vi "LoadDataLog.vi"(3 "entrée d'erreur":errorcluster, 4 "Shoot number to load":i32, 5 "Exp. folder":path) -> (0 "sortie d'erreur":errorcluster, 1 "Header Array":string[](array[string]), 2 "DataLoggingCluster":T1 {"Add. Param. No 2" format="%#_6f"; "Add. Param. No 1" format="%#_6f"; "Wedge Insertion (mm)" format="%#_6f"; "Pulse Duration (fs)" format="%#_6f"; "Parabola Position (um)" format="%#_6f"; "Pulse Energy (mJ)" format="%#_6f"; "Chirp (fs^2)" format="%#_6f"})   [LabVIEW 2014, in "ShhgDataLogging.lvlib"]
uses:
  ShhgDataLogging.lvlib
  DataLoggingCluster.ctl
panel:
  out "TimeString":string
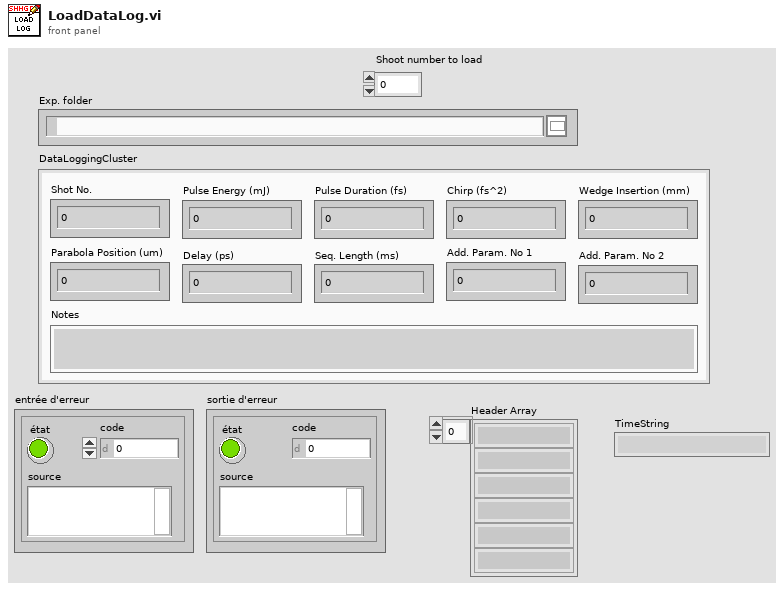
[diagram p1: front panel]
types:
  T1 = typedef "ShhgDataLogging.lvlib/DataLoggingCluster.ctl" = cluster{"Shot No. ":u32, "Pulse Energy (mJ)":dbl, "Pulse Duration (fs)":dbl, "Chirp (fs^2)":dbl, "Wedge Insertion (mm)":dbl, "Parabola Position (um)":dbl, "Delay (ps)":dbl, "Seq. Length (ms)":dbl, "Add. Param. No 1":dbl, "Add. Param. No 2":dbl, "Notes":string}
  T2 = enum16{"open", "replace", "create", "open or create", "replace or create", "replace or create with confirmation"}
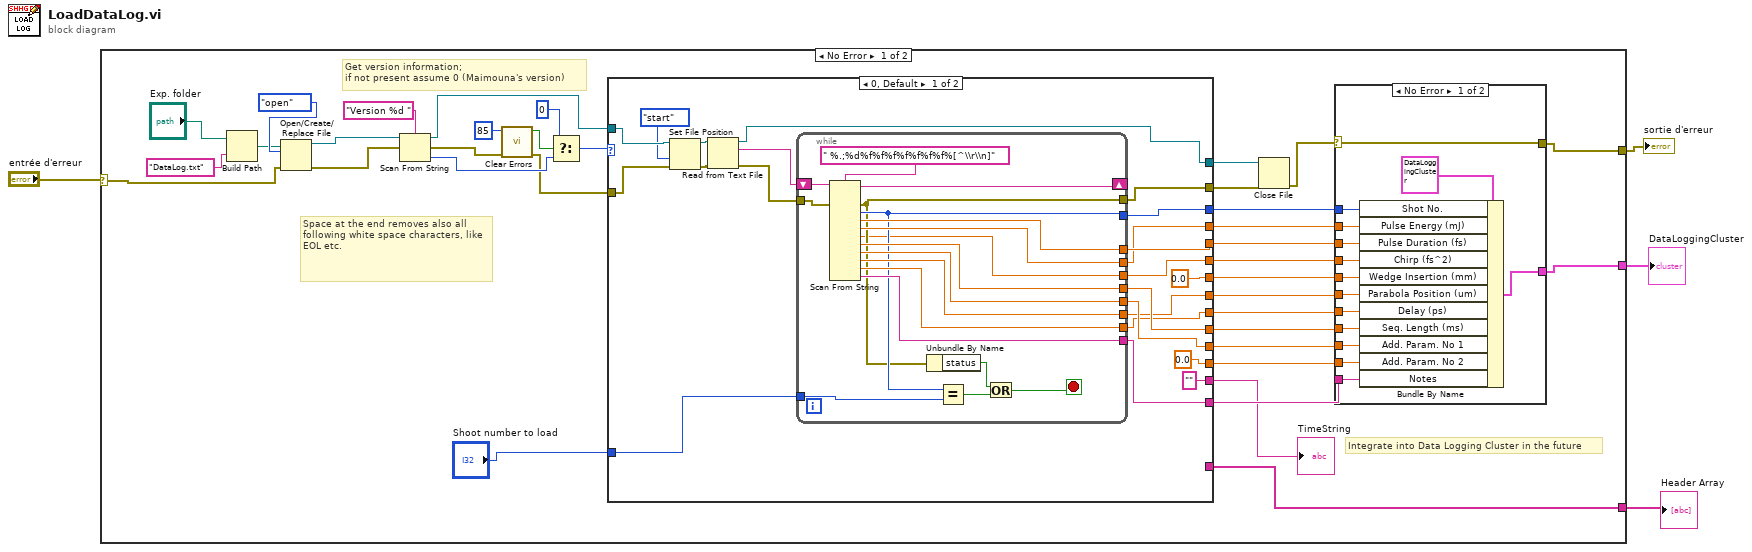
[diagram p0: block diagram]
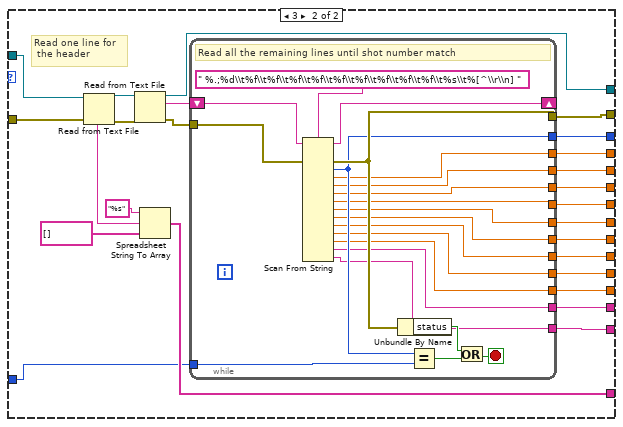
[diagram p2: hidden frame]
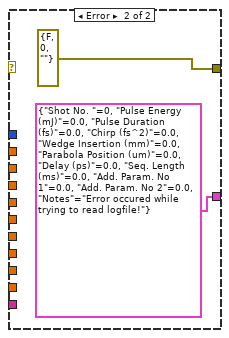
[diagram p3: hidden frame]
diagram:
  n1 = case shown="No Error" "entrée d'erreur" {
    selector: "entrée d'erreur" -> [w22 w142]
    tunnel: [w26 w142] -> w3
    tunnel: [w21 _] -> w2
    tunnel: [w6 _] -> w1
    frame No Error {
      # "Integrate into Data Logging Cluster in the future"
      # "Space at the end removes also all following white space characters, like EOL etc."
      # "Get version information; \nif not present assume 0 (Maimouna's version)"
      n2 = Build Path(base path="Exp. folder", name or relative path="DataLog.txt") -> (appended path=w23:path)
      n3 = Open/Create/Replace File(file path (use dialog)=w23, error in=w22, operation (0:open)=T2."open" ("opération (0 : open)")) -> (refnum out=w17:refnum<file>, error out=w11:errorcluster)  [unwired: 3 in, 1 out]
      n4 = Scan From String("Version %d " ("format string"), w17, w11) -> (w8:refnum<file>, w15:errorcluster, output 1=w12:i32)  [unwired: 1 in]
      n5 = call <vilib>:"Clear Errors.vi"("error in (no error)"=w15, "specific error code to clear (0: all)"=85) -> ("error out"=w10:errorcluster, "specific error cleared?"=w14:bool)  [unwired: 4 in]
      n6 = Select(t=0 ("specific error code to clear (0: all)"), s=w14, f=w12) -> (s? t:f=w9:i32)
      n7 = case shown="0, Default" w9 {
        tunnel: [w61 w98] -> w38
        tunnel: [w41 w82] -> w37
        tunnel: [w60 w87] -> w36
        tunnel: [w59 w86] -> w35
        tunnel: [w58 w88] -> w34
        tunnel: [w57 w92] -> w33
        tunnel: [w56 w93] -> w32
        tunnel: [w55 w90] -> w31
        tunnel: [w54 w95] -> w30
        tunnel: [w53 w96] -> w29
        tunnel: [w52 w91] -> w28
        tunnel: [0.0 ("Wedge Insertion (mm)") w89] -> w20
        tunnel: [0.0 ("Add. Param. No 2") w94] -> w19
        tunnel: w10 -> [w48 w103]
        tunnel: w8 -> [w49 w104]
        tunnel: [_ w99] -> w6
        tunnel: "Shoot number to load" -> [w46 w97]
        tunnel: ["" w80] -> w5
        frame 0, Default {
          n8 = Set File Position(refnum=w49, from (0:start)=enum16{"start", "end", "current"}."start", error in=w48) -> (refnum out=w45:refnum<file>, error out=w43:errorcluster)  [unwired: 1 in]
          n9 = Read from Text File(file (use dialog)=w45, error in=w43) -> (refnum out=w41:refnum<file>, text=w44:string, error out=w42:errorcluster)  [unwired: 2 in, 1 out]
          n10 = while {
            tunnel: [w66] -> w53
            tunnel: [w73] -> w54
            tunnel: [w67] -> w60
            tunnel: [w68] -> w59
            tunnel: [w64] -> w58
            tunnel: [w69] -> w57
            tunnel: [w70] -> w56
            tunnel: [w71] -> w55
            tunnel: [w72] -> w52
            tunnel: w46 -> [w74]
            shift-right: [w77] -> _
            shift-left: w44 -> [w63]
            tunnel: [w65] -> w61
            tunnel: w42 -> [w62]
            stop <- w75 stop-if-true
            n11 = Scan From String(format string=" %.;%d%f%f%f%f%f%f%f%[^\\r\\n]" ("chaîne de format"), input string=w63, error in=w62) -> (remaining string=w77:string, error out=w65:errorcluster, output 1=w66:i32, output 2=w67:dbl, output 3=w68:dbl, output 4=w64:dbl, output 5=w69:dbl, output 6=w70:dbl, output 7=w71:dbl, output 8=w72:dbl, output 9=w73:string)  [unwired: 10 in, 1 out]
            n12 = Unbundle By Name(w65) -> ("status"=w76:bool)
            n13 = Equal?(x=w66, y=w74) -> (x = y?=w78:bool)
            n14 = Or(x=w76, y=w78) -> (x .or. y?=w75:bool)
          }
        }
        frame 3 {
          # "Read one line for \n the header"
          n15 = Read from Text File(file (use dialog)=w104, error in=w103) -> (refnum out=w83:refnum<file>, text=w101:string, error out=w84:errorcluster)  [unwired: 2 in, 1 out]
          n16 = Read from Text File(file (use dialog)=w83, error in=w84) -> (refnum out=w82:refnum<file>, text=w81:string, error out=w85:errorcluster)  [unwired: 2 in, 1 out]
          n17 = Spreadsheet String To Array(format string="%s", spreadsheet string=w101, array type (2D Dbl)=string[] []) -> (array=w99:string[])  [unwired: 1 in]
          n18 = while {
            tunnel: w85 -> [w120]
            tunnel: [w117] -> w98
            tunnel: w97 -> [w122]
            tunnel: [w116] -> w96
            tunnel: [w106] -> w95
            tunnel: [w107] -> w94
            tunnel: [w108] -> w93
            tunnel: [w109] -> w92
            tunnel: [w110] -> w91
            tunnel: [w111] -> w90
            tunnel: [w112] -> w89
            tunnel: [w113] -> w88
            tunnel: [w114] -> w87
            tunnel: [w115] -> w86
            shift-right: [w119] -> _
            shift-left: w81 -> [w118]
            tunnel: [w105] -> w80
            stop <- w121 stop-if-true
            # "Read all the remaining lines until shot number match"
            n19 = Scan From String(format string=" %.;%d\\t%f\\t%f\\t%f\\t%f\\t%f\\t%f\\t%f\\t%f\\t%f\\t%s\\t%[^\\r\\n] ", input string=w118, error in=w120) -> (remaining string=w119:string, error out=w117:errorcluster, output 1=w116:i32, output 2=w115:dbl, output 3=w114:dbl, output 4=w113:dbl, output 5=w112:dbl, output 6=w111:dbl, output 7=w110:dbl, output 8=w109:dbl, output 9=w108:dbl, output 10=w107:dbl, output 11=w105:string, output 12=w106:string)  [unwired: 13 in, 1 out]
            n20 = Unbundle By Name(w117) -> ("status"=w124:bool)
            n21 = Equal?(x=w116, y=w122) -> (x = y?=w125:bool)
            n22 = Or(x=w124, y=w125) -> (x .or. y?=w121:bool)
          }
        }
      }
      "TimeString" <- w5
      n23 = Close File(refnum=w37, error in=w38) -> (error out=w27:errorcluster)  [unwired: 1 out]
      n24 = case shown="No Error" w27 {
        selector: w27 -> [w139 _]
        tunnel: [w130 T1 {"Shot No. "=0, "Pulse Energy (mJ)"=0.0, "Pulse Duration (fs)"=0.0, "Chirp (fs^2)"=0.0, "Wedge Insertion (mm)"=0.0, "Parabola Position (um)"=0.0, "Delay (ps)"=0.0, "Seq. Length (ms)"=0.0, "Add. Param. No 1"=0.0, "Add. Param. No 2"=0.0, "Notes"="Error occured while trying to read logfile!"} ("DataLoggingCluster 2")] -> w21
        tunnel: w36 -> [w128 _]
        tunnel: w35 -> [w129 _]
        tunnel: w34 -> [w136 _]
        tunnel: w33 -> [w133 _]
        tunnel: w32 -> [w132 _]
        tunnel: w31 -> [w135 _]
        tunnel: w30 -> [w131 _]
        tunnel: w29 -> [w137 _]
        tunnel: w28 -> [w134 _]
        tunnel: [w139 errorcluster {"status"=FALSE, "code"=0, "source"=""} ("error constant")] -> w26
        tunnel: w20 -> [w127 _]
        tunnel: w19 -> [w126 _]
        frame No Error {
          n25 = Bundle By Name(cluster=T1 {"Shot No. "=0, "Pulse Energy (mJ)"=0.0, "Pulse Duration (fs)"=0.0, "Chirp (fs^2)"=0.0, "Wedge Insertion (mm)"=0.0, "Parabola Position (um)"=0.0, "Delay (ps)"=0.0, "Seq. Length (ms)"=0.0, "Add. Param. No 1"=0.0, "Add. Param. No 2"=0.0, "Notes"=""} ("DataLoggingCluster 2"), "Shot No."=w137, "Pulse Energy (mJ)"=w129, "Pulse Duration (fs)"=w128, "Chirp (fs^2)"=w136, "Wedge Insertion (mm)"=w127, "Parabola Position (um)"=w135, "Delay (ps)"=w134, "Seq. Length (ms)"=w133, "Add. Param. No 1"=w132, "Add. Param. No 2"=w126, "Notes"=w131) -> (w130:T1)
        }
        frame Error {
        }
      }
    }
    frame Error {
    }
  }
  "sortie d'erreur" <- w3
  "DataLoggingCluster" <- w2
  "Header Array" <- w1
